vi "Test exception columns.vi"(11 "Test Case In":refnum<class "test Adjust Text to fit Rectangle.lvclass">) -> (0 "error out":errorcluster, 3 "Test Case Out":refnum<class "test Adjust Text to fit Rectangle.lvclass">)   [LabVIEW 2026, in "test Adjust Text to fit Rectangle.lvclass"]
uses:
  test Adjust Text to fit Rectangle.lvclass
  <vilib>/LabVIEW Icon API/API_Test Settings.ctl
  <vilib>/LabVIEW Icon API/lv_icon/Controls/Alignment.ctl
  <vilib>/LabVIEW Icon API/API_Text Colors.ctl
  <vilib>/LabVIEW Icon API/API_Text.ctl
  <vilib>/Astemes/LUnit/Test Case.lvclass/Test Case.ctl
  4993e8ee-a06a-463a-9684-69129f64d5ce.vi
  <vilib>/Astemes/LUnit/Core/LUnit Test Case/Private/Append Pass Result.vi
  <vilib>/Astemes/LUnit/Core/LUnit Test Case/Private/Append Fail Result.vi
  4993e8ee-a06a-463a-9684-69129f64d5ce.vi/9c5d11cd-9439-4240-a1ee-d9baace9c924.vi
  <vilib>/Astemes/LUnit/Core/LUnit Test Case/Private/Run In UI.vi
  <vilib>/Utility/error.llb/Clear Errors.vi
  test Adjust Text to fit Rectangle.lvclass/test Adjust Text to fit Rectangle.ctl
  <vilib>/LabVIEW Icon API/LabVIEW Icon API.lvlib
  <vilib>/LabVIEW Icon API/Set Text Icon/Text-Based VI Icon.lvlib
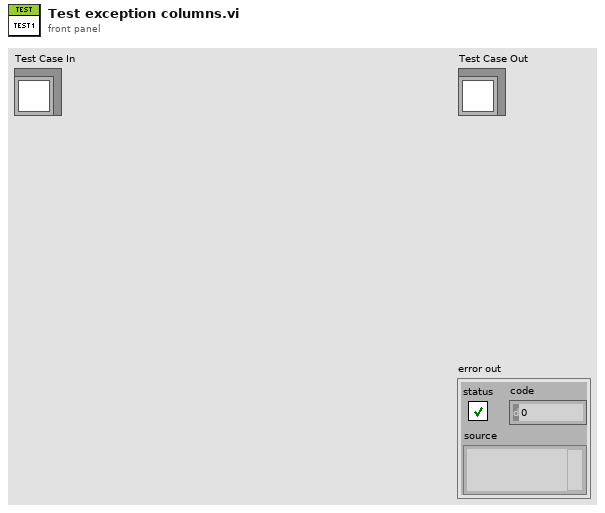
[diagram p1: front panel]
types:
  T1 = typedef "LabVIEW Icon API.lvlib/API_Text.ctl" = cluster{"Line 1 text":string, "Line 2 text":string, "Line 3 text":string, "Line 4 text":string}
  T2 = typedef "LabVIEW Icon API.lvlib/API_Test Settings.ctl" = cluster{"Font":string, "Alignment":T3, "Size":u8, "Center text":bool, "Capitalize text":bool, "Text color":T4}
  T3 = typedef "Alignment.ctl" = u16
  T4 = typedef "LabVIEW Icon API.lvlib/API_Text Colors.ctl" = cluster{"Line 1 color":u32, "Line 2 color":u32, "Line 3 color":u32, "Line 4 color":u32}
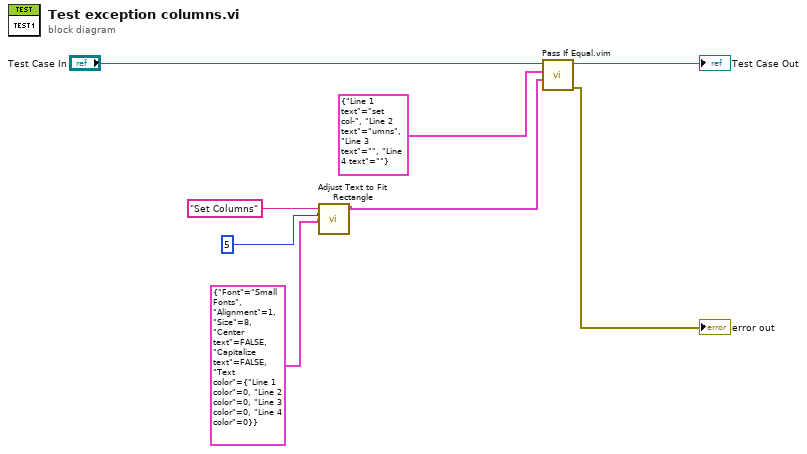
[diagram p0: block diagram]
diagram:
  n1 = call <vilib>:"Adjust Text to Fit Rectangle.vi"("VI Name"="Set Columns", "Number of Rows"=5, "Text settings"=T2 {"Font"="Small Fonts", "Alignment"=1, "Size"=8, "Center text"=FALSE, "Capitalize text"=FALSE, "Text color"={"Line 1 color"=0, "Line 2 color"=0, "Line 3 color"=0, "Line 4 color"=0}}) -> ("Text out"=w1:T1)  [unwired: 12 in]
  n2 = call "Pass If Equal.vim"("Actual"=w1, "Expected"=T1 {"Line 1 text"="set col-", "Line 2 text"="umns", "Line 3 text"="", "Line 4 text"=""} ("Text out"), "LUnit Test Case In"="Test Case In") -> ("error out"=→"error out":errorcluster, "LUnit Test Case Out"=→"Test Case Out":refnum<class "test Adjust Text to fit Rectangle.lvclass">)  [unwired: 7 in]
